vi "event_pairing_mode.vi"(5 "NewVal":bool, 7 "Ctrl Ref":refnum<vi>, 8 "error in":errorcluster, 9 "reference cluster in":T1) -> (0 "error out":errorcluster)   [LabVIEW 2016]
uses:
  Type Definitions/reference_cluster.ctl
  Type Definitions/vars_settings.ctl
  Type Definitions/stim_type.ctl
  Type Definitions/backlight_type.ctl
  Type Definitions/vars_runtime.ctl
  Type Definitions/data.ctl
  Type Definitions/notifier_elements_GUI.ctl
  Type Definitions/notifier_elements_DAQ.ctl
  Type Definitions/notifier_elements_write.ctl
  Type Definitions/control_references.ctl
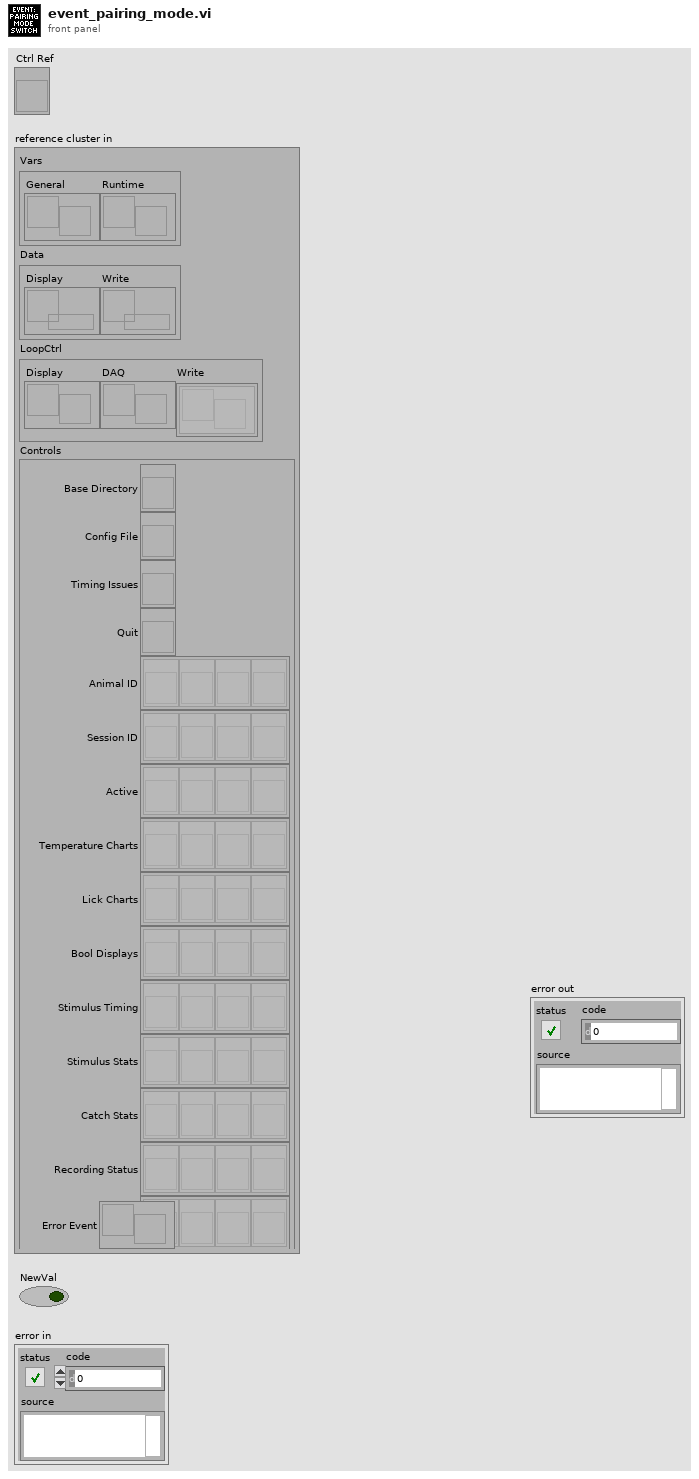
[diagram p1: front panel]
types:
  T1 = typedef "reference_cluster.ctl" = cluster{"Vars":cluster{"General":refnum<notifier>, "Runtime":refnum<notifier>}, "Data":cluster{"Display":refnum<queue>, "Write":refnum<queue>}, "LoopCtrl":cluster{"Display":refnum<notifier>, "DAQ":refnum<notifier>, "Write":refnum<notifier>[]}, "Controls":T2, "Error Event":refnum<user-event>}
  T2 = typedef "control_references.ctl" = cluster{"Base Directory":refnum<vi>, "Config File":refnum<vi>, "Timing Issues":refnum<vi>, "Quit":refnum<vi>, "Animal ID":refnum<vi>[], "Session ID":refnum<vi>[], "Active":refnum<vi>[], "Temperature Charts":refnum<vi>[], "Lick Charts":refnum<vi>[], "Bool Displays":refnum<vi>[], "Stimulus Timing":refnum<vi>[], "Stimulus Stats":refnum<vi>[], "Catch Stats":refnum<vi>[], "Recording Status":refnum<vi>[], "Pairing":refnum<vi>[]}
  T3 = typedef "vars_settings.ctl" = cluster{"base directory":path, "data directory":path, "active":bool, "running":bool, "pairing":bool, "clean tubes":bool, "animal ID":u16, "session ID":u16, "base temp":dbl, "d wait min":u16, "d wait max":u16, "d timeout":u16, "d reward":u16, "n reward":u16, "idx stim":u16, "timeout win":u16, "lick win":i32[], "stim type":T4[], "stim dur":u16[], "stim amp":dbl[], "stim freq":u16[], "stim ramp":u16[], "stim catch":u8[], "pairing delay":i16[], "square dur":u16[], "square delay":i16[], "square freq":u8[], "square dc":u8[], "stim shape":dbl[][], "square shape":bool[][], "backlight type":T5, "backlight freq":u16}
  T4 = typedef "stim_type.ctl" = enum16{"pulse", "vibration", "square", "sine"}
  T5 = typedef "backlight_type.ctl" = enum16{"none", "random", "regular"}
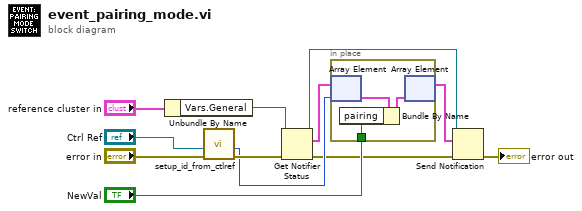
[diagram p0: block diagram]
diagram:
  n1 = Unbundle By Name("reference cluster in") -> ("Vars.General"=w9:refnum<notifier>)
  n2 = call "setup_id_from_ctlref.vi"("error in"="error in", "Ctl Refnum"="Ctrl Ref") -> ("error out"=w8:errorcluster, "setup ID"=w6:u16)  [unwired: 6 in]
  n3 = Get Notifier Status(notifier=w9, error in (no error)=w8) -> (notifier out=w5:refnum<notifier>, current notification=w4:T3[], error out=w2:errorcluster)  [unwired: 2 out]
  n4 = in-place {
    in-place-border: "NewVal" -> [w15]
    n5 = in-place-array #1(w4, w6) -> (w14:T3)
    n6 = Bundle By Name(cluster=w14, "pairing"=w15) -> (w13:T3)
    n7 = in-place-array #1(w13) -> (w3:T3[])  [unwired: 1 out]
  }
  n8 = Send Notification(notification=w3, notifier=w5, error in (no error)=w2) -> (error out=→"error out":errorcluster)  [unwired: 1 out]
